vi "LoadAndResizeImage.vi"(10 "Pixel Calibration Offset Image":path, 11 "Image in":T1) -> (1 "Valid":bool, 2 "Image as array":sgl[][](array[numeric]), 3 "Image out":T1)   [LabVIEW 2011]
uses:
  <vilib>/vision/Image Controls.llb/IMAQ Image.ctl
panel:
  out "Image":T1(plugin-control)
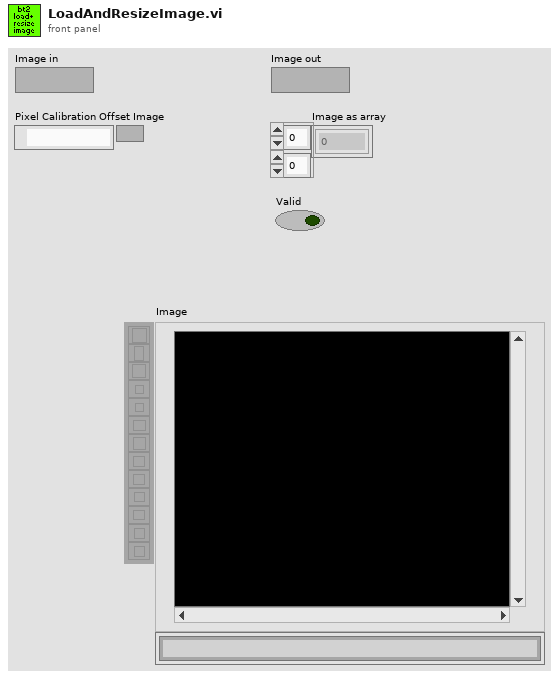
[diagram p1: front panel]
types:
  T1 = typedef "IMAQ Image.ctl" = refnum<image>
  T2 = enum16{"big-endian, network order", "native, host order", "little-endian"}
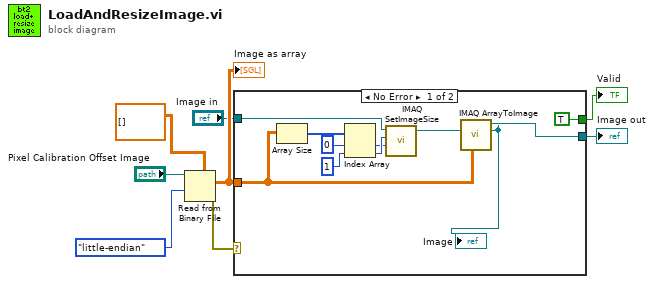
[diagram p0: block diagram]
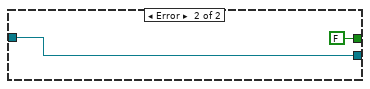
[diagram p2: hidden frame]
diagram:
  n1 = Read from Binary File(5:sgl[][] [], 9:T2."little-endian" ("byte order (0:big-endian, network order)"), 11:"Pixel Calibration Offset Image") -> (0:w5:errorcluster, 2:w6:sgl[][])  [unwired: 3 in, 2 out]
  "Image as array" <- w6
  n2 = case shown="No Error" w5 {
    tunnel: "Image in" -> [w16 w19]
    tunnel: [TRUE ("Use gain") FALSE ("Use gain")] -> w4
    tunnel: w6 -> [w15 _]
    tunnel: [w17 w19] -> w7
    frame No Error {
      n3 = Array Size(array=w15) -> (size(s)=w14:i32[])
      n4 = Index Array(array=w14, index #1=0 ("index"), index #2=1 ("index")) -> (element #1=w10:i32, element #2=w11:i32)
      n5 = call "IMAQ SetImageSize"("Y Resolution"=w10, "X Resolution"=w11, "Image"=w16) -> ("Image Out"=w9:T1)  [unwired: 2 in, 1 out]
      "Image" <- w9
      n6 = call "IMAQ ArrayToImage"("Image Pixels (Float)"=w15, "Image"=w9) -> ("Image Out"=w17:T1)  [unwired: 8 in, 1 out]
    }
    frame Error {
    }
  }
  "Image out" <- w7
  "Valid" <- w4
